vi "3.2.1-VectorNav Parse Reply.vi"(11 "Input String":string="$VNRRG,08,+000.00,+000.00,+000.00*00") -> (1 "Data":dbl[](array[numeric]), 2 "Register":T1, 3 "Header":string)   [LabVIEW 2010]
doc: "This VI parses the string reply from the VectorNav into usable data. The reply takes the form: \n\n$<Header>,<Register>,<Comma-delimited data>*<Checksum>\n\nThis VI looks at the header and register and saves the data in globals accordingly. For more specific information on the data, look at the VT-100 datasheet."
uses:
  3.2.1-VectorNav Registers.ctl
  <vilib>/regexp/Match Regular Expression.xnode
  _typedefs/3.2.1-VectorNav Data.ctl
  3.0-Global.vi
panel:
  out "Async Data Output Freq":dbl
  out "Async Data Output Type":dbl
  out "Serial Baud Rate":dbl
  out "Firmware Version":dbl
  out "Serial Number":dbl
  out "Hardware Revision":dbl
  out "Model":string
  out "Roll":dbl
  out "Pitch":dbl
  out "Yaw":dbl
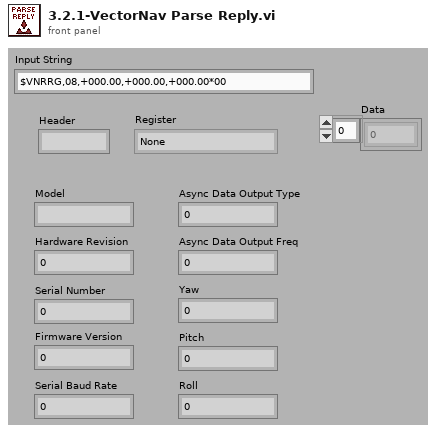
[diagram p1: front panel]
types:
  T1 = typedef "3.2.1-VectorNav Registers.ctl" = enum16{"None", "Model Number", "Hardware Revision", "Serial Number", "Firmware Version", "Serial Baud Rate", "Async Data Output Type", "Async Data Output Freq", "Attitude (Yaw, Pitch, Roll)", "Attitude (Quaternion)"}
  T2 = typedef "3.2.1-VectorNav Data.ctl" = cluster{"Yaw":dbl, "Pitch":dbl, "Roll":dbl}
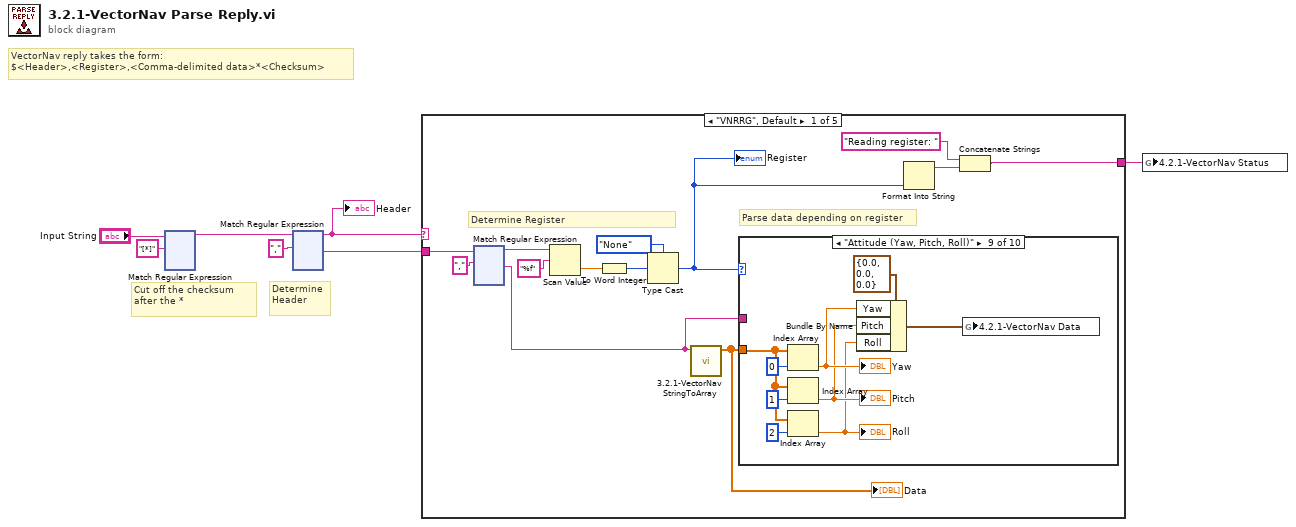
[diagram p0: block diagram]
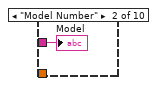
[diagram p3: hidden frame]
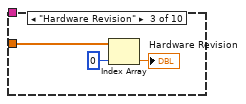
[diagram p4: hidden frame]
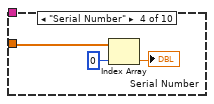
[diagram p5: hidden frame]
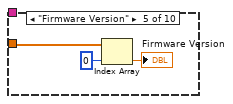
[diagram p6: hidden frame]
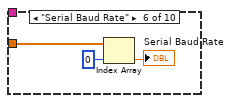
[diagram p7: hidden frame]
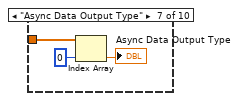
[diagram p8: hidden frame]
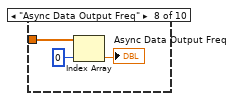
[diagram p9: hidden frame]
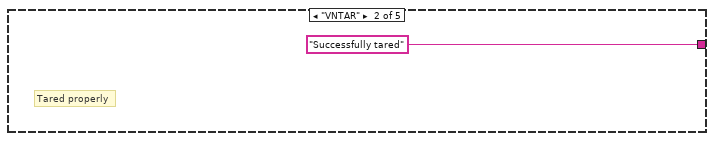
[diagram p11: hidden frame]
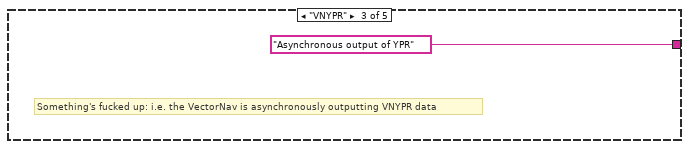
[diagram p12: hidden frame]
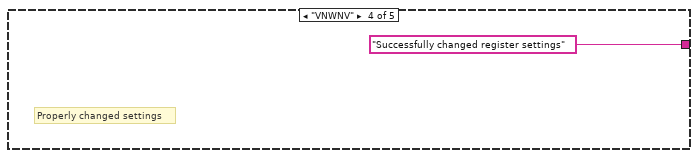
[diagram p13: hidden frame]
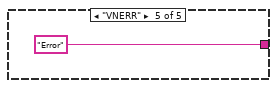
[diagram p14: hidden frame]
diagram:
  # "VectorNav reply takes the form:\n$<Header>,<Register>,<Comma-delimited data>*<Checksum>"
  # "Determine Header"
  # "Cut off the checksum after the *"
  n1 = xnode "Match Regular Expression"("input string"="Input String", "regular expression"="[*]") -> ("before match"=w3:string)  [unwired: 4 in, 4 out]
  n2 = xnode "Match Regular Expression"("input string"=w3, "regular expression"=",") -> ("before match"=w2:string, "after match"=w5:string)  [unwired: 4 in, 3 out]
  "Header" <- w2
  n3 = case shown="\"VNRRG\", Default" w2 {
    tunnel: w5 -> [w18 _ _ _ _]
    tunnel: [w8 "Successfully tared" "Asynchronous output of YPR" "Successfully changed register settings" "Error"] -> w1
    frame "VNRRG", Default {
      # "Parse data depending on register"
      # "Determine Register"
      n4 = xnode "Match Regular Expression"("input string"=w18, "regular expression"=",") -> ("before match"=w12:string, "after match"=w13:string)  [unwired: 4 in, 3 out]
      n5 = Scan Value(string=w12, format string="%f") -> (value=w15:dbl)  [unwired: 1 in, 1 out]
      n6 = To Word Integer(number=w15) -> (16bit integer=w16:i16)
      n7 = Type Cast(type=3.2.1-VectorNav_Registers."None" ("VectorNav Registers"), x=w16) -> (*(type *) &x=w9:T1)
      "Register" <- w9
      n8 = call "3.2.1-VectorNav StringToArray.vi"("String"=w13) -> ("Array"=w14:dbl[])  [unwired: 10 in]
      "Data" <- w14
      n9 = case shown="\"Attitude (Yaw, Pitch, Roll)\"" w9 {
        tunnel: w13 -> [_ w21 _ _ _ _ _ _ _ _]
        tunnel: w14 -> [_ _ w22 w25 w28 w31 w34 w37 w45 _]
        frame "None", Default {
        }
        frame "Model Number" {
          "Model" <- w21
        }
        frame "Hardware Revision" {
          n10 = Index Array(array=w22, index=0) -> (element=→"Hardware Revision":dbl)
        }
        frame "Serial Number" {
          n11 = Index Array(array=w25, index=0) -> (element=→"Serial Number":dbl)
        }
        frame "Firmware Version" {
          n12 = Index Array(array=w28, index=0) -> (element=→"Firmware Version":dbl)
        }
        frame "Serial Baud Rate" {
          n13 = Index Array(array=w31, index=0) -> (element=→"Serial Baud Rate":dbl)
        }
        frame "Async Data Output Type" {
          n14 = Index Array(array=w34, index=0) -> (element=→"Async Data Output Type":dbl)
        }
        frame "Async Data Output Freq" {
          n15 = Index Array(array=w37, index=0) -> (element=→"Async Data Output Freq":dbl)
        }
        frame "Attitude (Yaw, Pitch, Roll)" {
          n16 = Index Array(array=w45, index=0) -> (element=w42:dbl)
          "Yaw" <- w42
          n17 = Index Array(array=w45, index=1) -> (element=w41:dbl)
          "Pitch" <- w41
          n18 = Index Array(array=w45, index=2) -> (element=w40:dbl)
          "Roll" <- w40
          n19 = Bundle By Name(cluster=T2 {"Yaw"=0.0, "Pitch"=0.0, "Roll"=0.0} ("VectorNav Data"), "Yaw"=w42, "Pitch"=w41, "Roll"=w40) -> (w44:T2)
          n20 = global write "3.0-Global.vi" "4.2.1-VectorNav Data"(w44) -> ()
        }
        frame "Attitude (Quaternion)" {
        }
      }
      n21 = Format Into String(w9) -> (resulting string=w10:string)  [unwired: 3 in, 1 out]
      n22 = Concatenate Strings("Reading register: " ("4.1.1-VectorNav Status"), w10) -> (w8:string)
    }
    frame "VNTAR" {
      # "Tared properly"
    }
    frame "VNYPR" {
      # "Something's fucked up: i.e. the VectorNav is asynchronously outputting VNYPR data"
    }
    frame "VNWNV" {
      # "Properly changed settings"
    }
    frame "VNERR" {
    }
  }
  n23 = global write "3.0-Global.vi" "4.2.1-VectorNav Status"(w1) -> ()
